vi "Do That Thang.vi"(8 "error in (no error)":errorcluster, 9 "Lookup Table":refnum<data-value>, 11 "Parallelizer in":refnum<class "Parallelizer.lvclass">) -> (0 "error out":errorcluster, 3 "Parallelizer out":refnum<class "Parallelizer.lvclass">)   [LabVIEW 2019, in "Parallelizer Example.lvlib" / "Parallelizer.lvclass"]
uses:
  <vilib>/gpm_packages/@cs/test-executive/Source/Sandbox/Parallelizer Example/Parallelizer/Parallelizer.lvclass
  C:/Program Files/National Instruments/LabVIEW 2019/vi.lib/ActorFramework/Actor/Actor.lvclass
  <vilib>/gpm_packages/@cs/lookup-table/Source/LookupTable/LookupTable.lvclass
  <vilib>/gpm_packages/@cs/test-executive/Source/Sandbox/Parallelizer Example/Process Model/Process Model.lvclass
  <vilib>/gpm_packages/@cs/test-executive/Source/Sandbox/Parallelizer Example/Parallelizer/Parallelizer.lvclass/Parallelizer.ctl
  <vilib>/gpm_packages/@cs/test-executive/Source/Sandbox/Parallelizer Example/Process Model/Process Model.lvclass/Process Model.ctl
  <vilib>/gpm_packages/@cs/test-executive/Source/Sandbox/Parallelizer Example/Process Model Messages/Create Process Msg/Create Process Msg.lvclass/Create Process Msg.ctl
  <vilib>/ActorFramework/Message Enqueuer/Message Enqueuer.lvclass/Message Enqueuer.ctl
  <vilib>/ActorFramework/Message Enqueuer/Enqueue.vi
  <vilib>/gpm_packages/@cs/test-executive/Source/Sandbox/Parallelizer Example/Process Model Messages/Create Process Msg/Create Process Msg.lvclass
  C:/Program Files/National Instruments/LabVIEW 2019/vi.lib/ActorFramework/Message/Message.lvclass
  <vilib>/ActorFramework/Message Priority Queue/Priority Enqueue.vi
  <vilib>/ActorFramework/Actor/Actor.lvclass
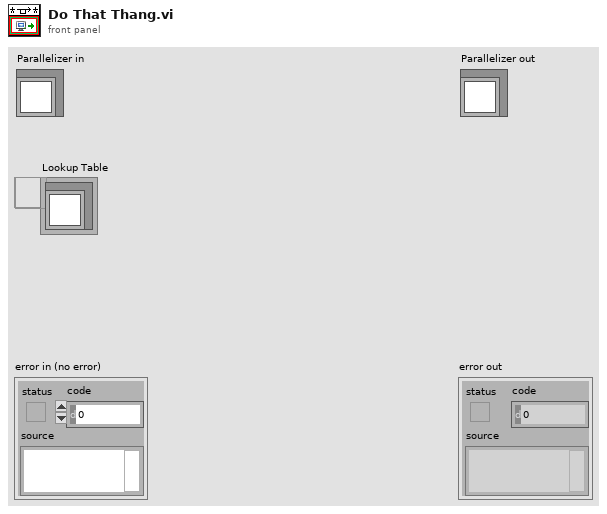
[diagram p1: front panel]
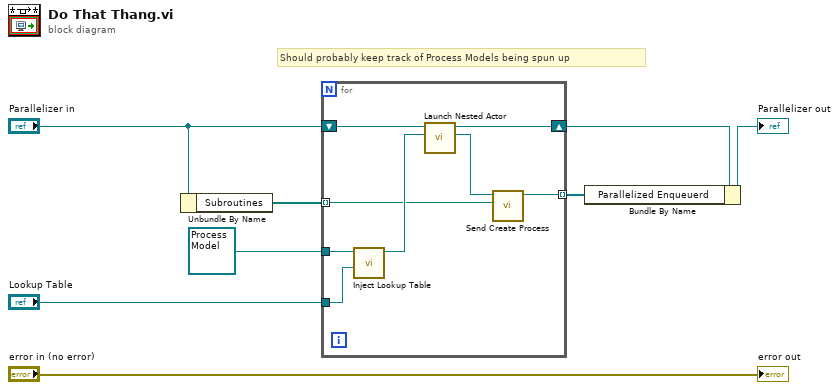
[diagram p0: block diagram]
diagram:
  # "Should probably keep track of Process Models being spun up"
  n1 = Unbundle By Name("Parallelizer in") -> ("Subroutines"=w7:path[])
  n2 = for {
    tunnel: w7 -> [w10] mode=indexing
    tunnel: refnum<class "Process Model.lvclass"> refnum ("Parallelizer Example.lvlib:Process Model.lvclass") -> [w14]
    tunnel: "Lookup Table" -> [w12]
    shift-right: [w15] -> w3
    shift-left: "Parallelizer in" -> [w16]
    tunnel: [w9] -> w1 mode=indexing
    n3 = call <vilib>:"Inject Lookup Table.vi"("LookupTable"=w12, "Process Model in"=w14) -> ("Process Model out"=w13:refnum<class "Process Model.lvclass">)  [unwired: 9 in]
    n4 = call <vilib>:"Launch Nested Actor.vi"("Nested Actor"=w13, "Caller Actor in"=w16) -> ("Nested Actor's Enqueuer"=w11:refnum<class "Message Enqueuer.lvclass">, "Caller Actor out"=w15:refnum<class "Parallelizer.lvclass">)  [unwired: 7 in, 1 out]
    n5 = call <vilib>:"Send Create Process.vi"("Subroutine"=w10, "Message Enqueuer"=w11) -> ("Message Enqueuer out"=w9:refnum<class "Message Enqueuer.lvclass">)  [unwired: 8 in, 1 out]
  }
  n6 = Bundle By Name(cluster=w3, "Parallelized Enqueuerd"=w1) -> (→"Parallelizer out":refnum<class "Parallelizer.lvclass">)
  "error out" <- "error in (no error)"
